vi "variantTypeToFloat.vi"(10 "variant":variant, 11 "Type In":i16[](array[numeric])) -> (2 "Double":dbl, 3 "Type Out":i16[](array[numeric]))   [LabVIEW 2011]
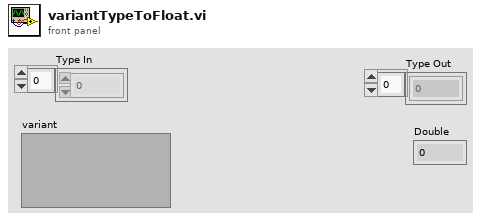
[diagram p1: front panel]
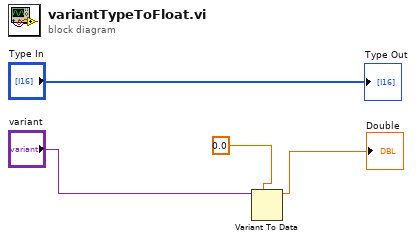
[diagram p0: block diagram]
diagram:
  n1 = Variant To Data(type=0.0, Variant="variant") -> (data=→"Double":dbl)  [unwired: 1 in, 1 out]
  "Type Out" <- "Type In"
